vi "MercuryITC-VISA-write.vi"(8 "error in (no error)":errorcluster, 10 "write buffer":string, 11 "VISA resource name":refnum<visa-resource-name>) -> (0 "error out":errorcluster, 2 "read buffer":string, 3 "VISA resource name out":refnum<visa-resource-name>)   [LabVIEW 2012]
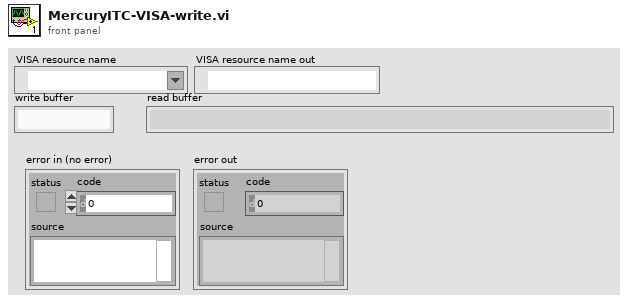
[diagram p1: front panel]
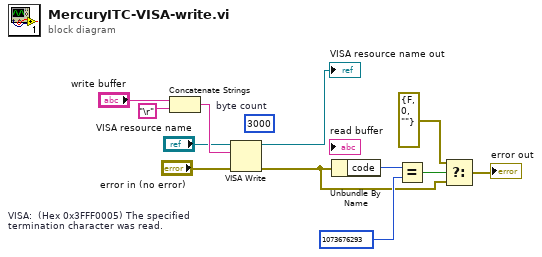
[diagram p0: block diagram]
diagram:
  w8 = 1073676293  # VISA:  (Hex 0x3FFF0005) The specified termination character was read.
  (unwired) u32 3000  # byte count
  n1 = Concatenate Strings("write buffer", "\r") -> (w11:string)
  n2 = VISA Write(VISA resource name="VISA resource name", write buffer=w11, error in (no error)="error in (no error)") -> (VISA resource name out=→"VISA resource name out":refnum<visa-resource-name>, error out=w2:errorcluster)  [unwired: 1 out]
  n3 = Unbundle By Name(w2) -> ("code"=w9:i32)
  n4 = Equal?(x=w9, y=w8) -> (x = y?=w6:bool)
  n5 = Select(t=errorcluster {"status"=FALSE, "code"=0, "source"=""}, s=w6, f=w2) -> (s? t:f=→"error out":errorcluster)
